vi "Delete Doc by Index.vi"(8 "error in (no error)":errorcluster, 10 "Doc index[]":i32[](array[numeric]), 11 "LV MDI in":refnum<class "LV MDI.lvclass">) -> (0 "error out":errorcluster, 3 "LV MDI out":refnum<class "LV MDI.lvclass">)   [LabVIEW 2016, in "LV MDI.lvclass"]
uses:
  LV MDI.lvclass
  LV MDI.lvclass/LV MDI.ctl
  Document/Document base/Document.lvclass
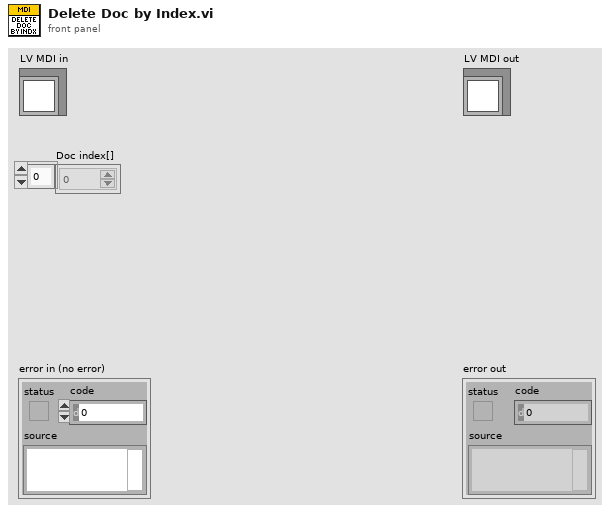
[diagram p1: front panel]
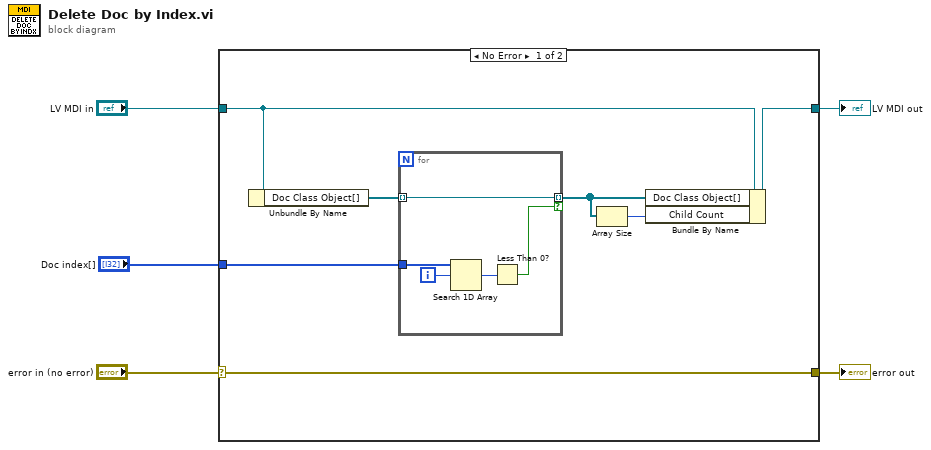
[diagram p0: block diagram]
diagram:
  n1 = case shown="No Error" "error in (no error)" {
    selector: "error in (no error)" -> [w12 w19]
    tunnel: [w12 w19] -> w4
    tunnel: [w8 w18] -> w2
    tunnel: "LV MDI in" -> [w9 w18]
    tunnel: "Doc index[]" -> [w11 _]
    frame No Error {
      n2 = Unbundle By Name(w9) -> ("Doc Class Object[]"=w10:refnum<class "Document.lvclass">[])
      n3 = for {
        tunnel: w11 -> [w16]
        tunnel: w10 -> [w17] mode=indexing
        tunnel: [w17] -> w6 mode=indexing if=w13
        i -> [w15]
        n4 = Search 1D Array(1D array=w16, element=w15) -> (index of element=w14:i32)  [unwired: 1 in]
        n5 = Less Than 0?(x=w14) -> (x < 0?=w13:bool)
      }
      n6 = Array Size(array=w6) -> (size(s)=w7:i32)
      n7 = Bundle By Name(cluster=w9, "Doc Class Object[]"=w6, "Child Count"=w7) -> (w8:refnum<class "LV MDI.lvclass">)
    }
    frame Error {
    }
  }
  "error out" <- w4
  "LV MDI out" <- w2
